vi "Bytes to word.vi"(5 "Litt/BigEnd":bool, 7 "Index":i32, 8 "Image Data in":u8[](array[numeric])) -> (1 "Index+2":i32, 2 "Word":u16)   [LabVIEW 2013, in "Tiff reader.lvlib"]
doc: "This .vi converts 2bytes to a word.\n\n(Inlined to prevent array extra copies)"
uses:
  Tiff reader.lvlib
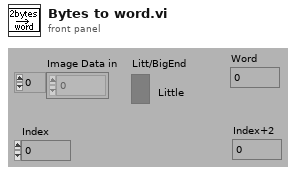
[diagram p1: front panel]
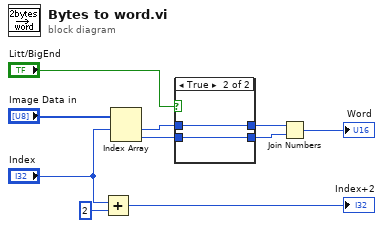
[diagram p0: block diagram]
diagram:
  n1 = Add(x="Index", y=2) -> (x+y=→"Index+2":i32)
  n2 = Index Array(array="Image Data in", index #1="Index") -> (element #1=w8:u8, element #2=w7:u8)  [unwired: 1 in]
  n3 = case shown="True" "Litt/BigEnd" {
    tunnel: w8 -> [w11 w14]
    tunnel: [w12 w14] -> w5
    tunnel: w7 -> [w12 w13]
    tunnel: [w11 w13] -> w6
    frame False {
    }
    frame True {
    }
  }
  n4 = Join Numbers(hi=w5, lo=w6) -> ((hi.lo)=→"Word":u16)
